vi "Data Archiving.vi"() -> ()   [LabVIEW 2009]
uses:
  lib/Apps/App Status Actions.ctl
  lib/Data Access Objects/Metadata/Persistant DAO Actions.ctl
  lib/Logging/LogFileType.ctl
  lib/MixedMode/Mixed Mode States.ctl
  lib/Launcher/Launcher Actions.ctl
  lib/Launcher/NoPanelAppTypes.ctl
  lib/Data Access Objects/Metadata/DAO Actions.ctl
  lib/MixedMode/Mixed Mode Archived State.ctl
  lib/Apps/Yes No Button.ctl
  lib/Global Data/Transactions/Dataset Type.ctl
  lib/Global Data/Transactions/Dataset Source.ctl
  lib/Global Data/Transactions/Dataset Transaction Id.ctl
  lib/Logging/Command or Stiffness Updates.ctl
  lib/Global Data/Jacobian Stiffness Column Id.ctl
  lib/Global Data/Jacobian Stiffness Column.ctl
  lib/MixedMode/Target Data.ctl
  lib/Global Data/Command Or Stiffness Update Type.ctl
  lib/Logging/Command or Stiffnness Record.ctl
  lib/Logging/Archive File Type.ctl
panel:
  out "current time":timestamp
  out "Step":string
  out "all stopped":bool
  out "Continuous Archive Buffer Size":i32(slide) scale=0.0..1000.0
  out "MixedModeStates":T1
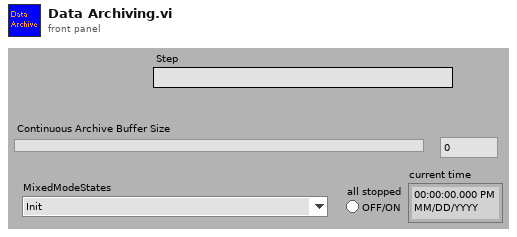
[diagram p1: front panel]
types:
  T1 = typedef "Mixed Mode States.ctl" = enum16{"Init", "Wait For DAQ", "Idle", "Start Initial Position", "Initial Position", "Start Initial Ramp", "Run Initial Ramp", "Start Iterative Stage", "Convergence Check", "Update Stiffness Jacobian", "Update Command", "Start Iterative Ramp", "Run Iterative Ramp", "Start Iterative Stabilize", "Iterative Stabilize", "Start Iterative Holding", "Iterative Holding", "Start Stabilize", "Stabilize", "Start Hold", "Holding", "Done", "Aborting", "Exit", "Nop"}
  T2 = typedef "Command or Stiffnness Record.ctl" = cluster{"Command || Stiffness Update":T3, "Records":string[]}
  T3 = typedef "Command or Stiffness Updates.ctl" = enum16{"Command Update", "Iterative Command Update", "Stiffness Update"}
  T4 = typedef "Command Or Stiffness Update Type.ctl" = cluster{"Target":T5[], "Stiffness":T6[], "Command || Stiffness Update":T3}
  T5 = typedef "Target Data.ctl" = cluster{"Displacements":dbl[], "Command Type":enum16{"<None>", "Displacement", "Force"}[], "Forces":dbl[]}
  T6 = typedef "Jacobian Stiffness Column.ctl" = cluster{"Id":T7, "Column":dbl[]}
  T7 = typedef "Jacobian Stiffness Column Id.ctl" = enum16{"dDx", "dDy", "dDz", "dRx", "dRy", "dRz"}
  T8 = typedef "Dataset Transaction Id.ctl" = cluster{"Dataset Source":T9, "Dataset Type":T10, "Hold":T11, "Volts":T11, "Tag":string}
  T9 = typedef "Dataset Source.ctl" = enum16{"LBCB 1", "LBCB 2", "Combined", "External Sensors"}
  T10 = typedef "Dataset Type.ctl" = enum16{"LVDT", "Load Cell", "Actuator Command", "Servo Error", "Displacement Command", "Displacement", "Force"}
  T11 = typedef "Yes No Button.ctl" = bool
  T12 = typedef "Mixed Mode Archived State.ctl" = cluster{"MixedModeStates":T1, "Step":string}
  T13 = typedef "Persistant DAO Actions.ctl" = enum16{"Init", "Get", "Set", "Load", "Save"}
  T14 = typedef "DAO Actions.ctl" = enum16{"Init", "Get", "Set"}
  T15 = typedef "Number Of LBCBs.ctl" = enum16{"1", "2"}
  T16 = typedef "App Parameters.ctl" = cluster{"Monitor Loop":T17, "Ramp Time":T17, "Log Loop":T17, "TCP to DAQ":T17, "Logging Directory":path, "Log File Size (MBytes)":i64, "Volt Logging Loop":T17, "2 LBCB Archiving Mode":bool}
  T17 = typedef "Timing Parameters.ctl" = cluster{"Interval":dbl, "Rate ":dbl}
  T18 = typedef "Archive File Type.ctl" = enum16{"LBCB1", "LBCB2", "ExternalSensors", "Combined"}
  T19 = typedef "App Status Actions.ctl" = enum16{"Init", "Get Status", "Running", "Control", "Autobalanced", "Data Acquisition", "Set App State", "DAQ Started", "Set LBCB State", "Set All", "Set Cont Logging", "Set Step Logging", "Set MM Logging", "Set Volt Logging", "Set DAQ Link"}
  T20 = typedef "LogFileType.ctl" = enum16{"Continuous", "Step", "Volts", "Offsets", "DLL  Errors", "Snapshot", "Commands", "StiffnessUpdates", "End List"}
  T21 = typedef "App Status.ctl" = cluster{"Running":bool, "Controlling L2":bool, "Autobalance L2":bool, "Data Acquisition":bool, " App State":T22, "DAQ Started":bool, "LBCB 1 State":T23, "LBCB 2 State":T23, "Controlling L1":bool, "Autobalance L1":bool, "Continuous Logging":bool, "Step Logging":bool, "Voltage Logging":bool, "Mixed Mode Logging":bool, "DAQ Link":bool}
  T22 = typedef "AppStates.ctl" = enum16{"Starting OM", "Initializing Displays", "Setting up Archiving", "Setting Up DAQ Channels", "Start DAQ", "DAQ Starting", "Controlling LBCBs", "Stopping OM"}
  T23 = typedef "Lbcb Control Loop States.ctl" = enum16{"Idle", "Start Selected", "Load Last Command", "Start Autobalancing", "Autobalancing", "Control Loop Initialized", "Control Enabled"}
  T24 = typedef "Network Parameters.ctl" = cluster{"Port Number":u16, "Notification Name":string, "Wait For Notification Timeout":i32}
  T25 = typedef "NoPanelAppTypes.ctl" = enum16{"NTCP Socket", "Data Archiving", "DAQ Link", "Control Loops", "Cmd Disp Diffs", "LBCB Data", "Limits", "Mixed Mode Widget", "Offsets"}
  T26 = typedef "Launcher Actions.ctl" = enum16{"Launch", "Stop All", "Stop", "Kill", "Running?", "Init"}
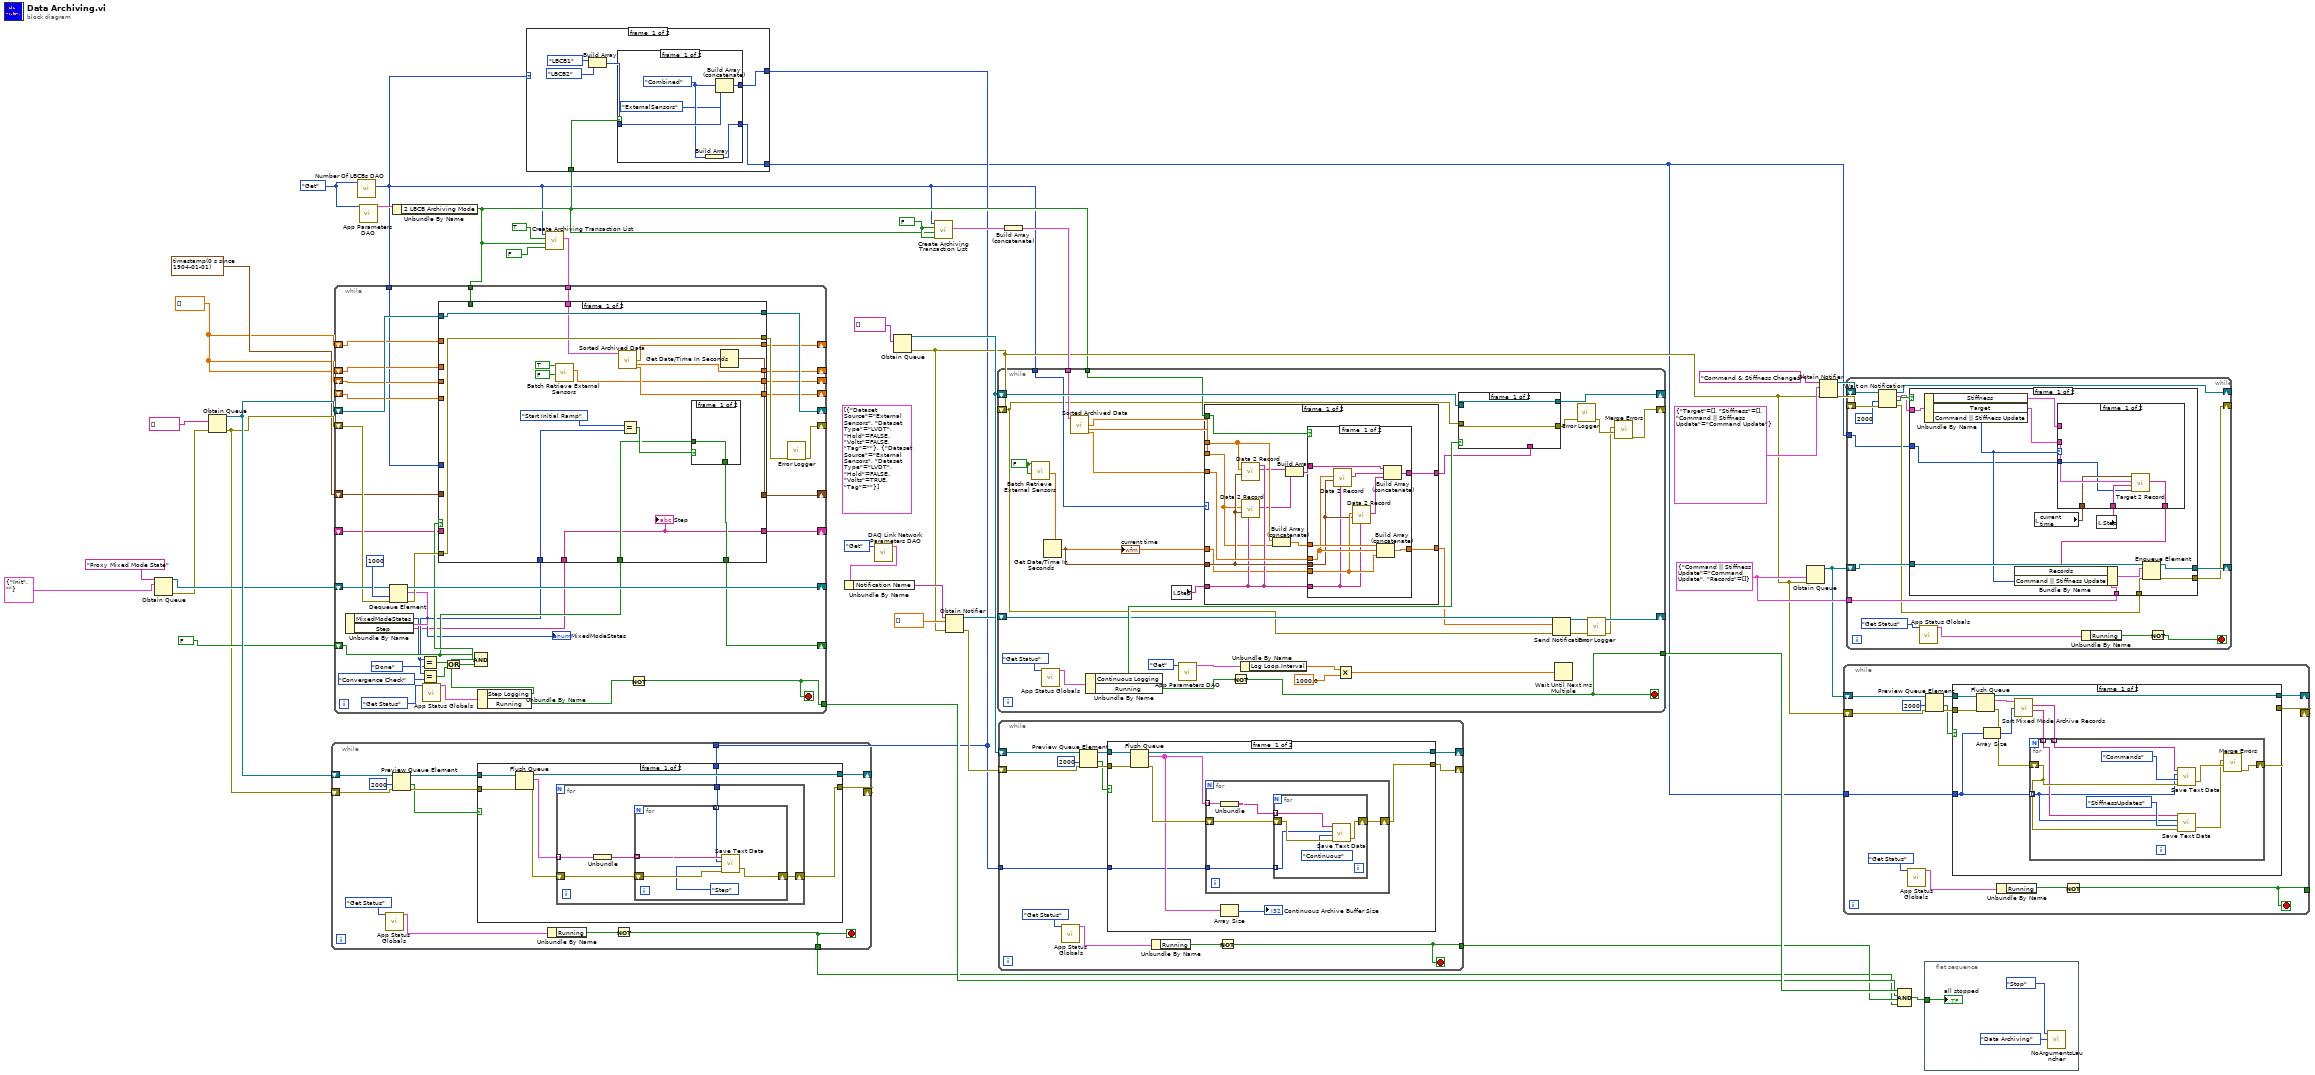
[diagram p0: block diagram]
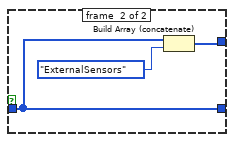
[diagram p2: hidden frame]
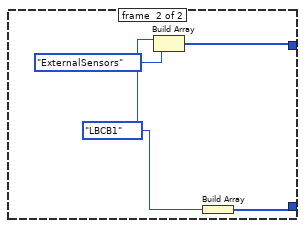
[diagram p3: hidden frame]
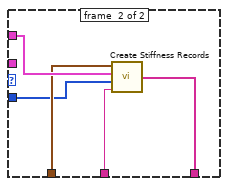
[diagram p5: hidden frame]
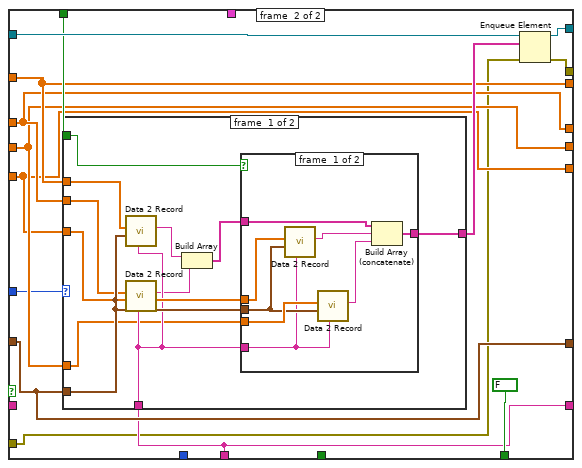
[diagram p9: hidden frame]
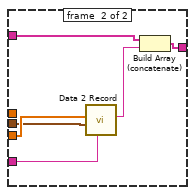
[diagram p10: hidden frame]
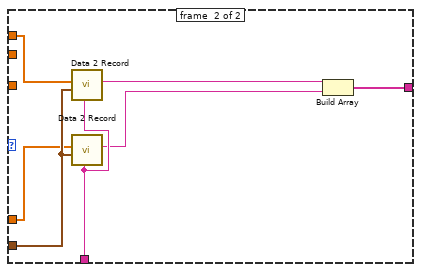
[diagram p11: hidden frame]
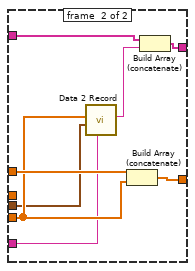
[diagram p13: hidden frame]
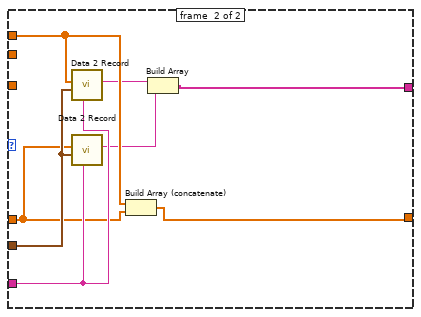
[diagram p14: hidden frame]
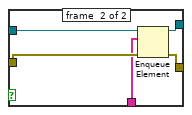
[diagram p15: hidden frame]
diagram:
  w7 = T2 {"Command || Stiffness Update"=enum."Command Update", "Records"=[]} ("Command || Stiffness Record")
  (unwired) T8[] [{"Dataset Source"=enum."External Sensors", "Dataset Type"=enum."LVDT", "Hold"=FALSE, "Volts"=FALSE, "Tag"=""}, {"Dataset Source"=enum."External Sensors", "Dataset Type"=enum."LVDT", "Hold"=FALSE, "Volts"=TRUE, "Tag"=""}] ("Transactions")
  w14 = T11 FALSE ("Hold")
  w21 = Persistant_DAO_Actions."Get" ("Actions")
  w25 = dbl[] [] ("Data")
  n1 = Obtain Queue(name (unnamed)="Proxy Mixed Mode State", element data type=T12 {"MixedModeStates"=enum."Init", "Step"=""} ("Mixed Mode Archived State")) -> (queue out=w38:refnum<queue>, error out=w37:errorcluster)  [unwired: 3 in, 1 out]
  n2 = Obtain Queue(element data type=string[] [] ("Records"), error in (no error)=w37) -> (queue out=w40:refnum<queue>, error out=w33:errorcluster)  [unwired: 2 in, 2 out]
  n3 = call "Number Of LBCBs DAO.vi"("Actions"=w21) -> ("Number of\nLBCBs Out"=w2:T15)  [unwired: 7 in, 3 out]
  n4 = call "App Parameters DAO.vi"("Actions"=w21) -> ("Application Timing and Logging Out"=w20:T16)  [unwired: 8 in, 2 out]
  n5 = Unbundle By Name(w20) -> ("2 LBCB Archiving Mode"=w4:bool)
  n6 = case shown="\"2\"" w2 {
    tunnel: w4 -> [w48 _]
    tunnel: [w44 w58] -> w3
    tunnel: [w43 w57] -> w1
    frame #0 {
      n7 = Build Array(Archive_File_Type."LBCB1" ("Archive File Type"), Archive_File_Type."LBCB2" ("element")) -> (w46:T18[])
      n8 = case shown="True" w48 {
        tunnel: w46 -> [w53 w56]
        tunnel: [w50 w54] -> w44
        tunnel: [w49 w56] -> w43
        frame #0 {
          w52 = Archive_File_Type."Combined" ("element")
          n9 = Build Array(w52) -> (w49:T18[])
          n10 = Build Array (concatenate)(w53, w52, Archive_File_Type."ExternalSensors" ("element")) -> (w50:T18[])
        }
        frame #1 {
          n11 = Build Array (concatenate)(w56, Archive_File_Type."ExternalSensors" ("element")) -> (w54:T18[])
        }
      }
    }
    frame #1 {
      w60 = Archive_File_Type."LBCB1" ("Archive File Type")
      n12 = Build Array(w60, Archive_File_Type."ExternalSensors" ("element")) -> (w58:T18[])
      n13 = Build Array(w60) -> (w57:T18[])
    }
  }
  n14 = while {
    shift-right: [w64] -> _
    shift-left: w40 -> [w67]
    shift-right: [w65] -> _
    shift-left: w33 -> [w66]
    tunnel: [w62] -> w29
    tunnel: w3 -> [w61]
    stop <- w62 stop-if-true
    n15 = call "App Status Globals.vi"("App Status Actions"=App_Status_Actions."Get Status") -> ("App Status Out"=w72:T21)  [unwired: 5 in, 9 out]
    n16 = Preview Queue Element(queue=w67, timeout in ms (-1)=2000, error in (no error)=w66) -> (queue out=w68:refnum<queue>, timed out?=w63:bool, error out=w69:errorcluster)  [unwired: 1 out]
    n17 = case shown="False" w63 {
      tunnel: w68 -> [w80 w92]
      tunnel: w69 -> [w79 w91]
      tunnel: [w78 w92] -> w64
      tunnel: [w76 w91] -> w65
      tunnel: w61 -> [w74 _]
      frame #0 {
        n18 = Flush Queue(queue=w80, error in (no error)=w79) -> (queue out=w78:refnum<queue>, remaining elements=w75:cluster{"Records":string[]}[], error out=w77:errorcluster)
        n19 = for {
          tunnel: w75 -> [w83] mode=indexing
          shift-right: [w84] -> w76
          shift-left: w77 -> [w85]
          tunnel: w74 -> [w81]
          n20 = Unbundle(w83) -> ("Records"=w82:string[])
          n21 = for {
            shift-right: [w88] -> w84
            shift-left: w85 -> [w90]
            tunnel: w82 -> [w87] mode=indexing
            tunnel: w81 -> [w86] mode=indexing
            n22 = call "Save Text Data.vi"("String"=w87, "Archive File Type"=w86, "LogFile Type"=LogFileType."Step", "error in"=w90) -> ("error out"=w88:errorcluster)  [unwired: 1 in, 1 out]
          }
        }
      }
      frame #1 {
      }
    }
    n23 = Unbundle By Name(w72) -> ("Running"=w73:bool)
    n24 = Not(x=w73) -> (.not. x?=w62:bool)
  }
  n25 = call "Create Archiving Transaction List.vi"("Volts Only"=FALSE ("Include Volts"), "Combined LBCBs"=w4, "Hold"=T11 TRUE, "Number of LBCBs"=w2) -> ("Transactions"=w15:T8[])  [unwired: 7 in]
  n26 = while {
    shift-right: [w128] -> _
    shift-left: w40 -> [w129]
    shift-right: [w126] -> _
    shift-left: w33 -> [w122]
    shift-right: [w123] -> _
    shift-left: w38 -> [w124]
    shift-right: [w118] -> _
    shift-left: FALSE -> [w115]
    tunnel: [w116] -> w31
    shift-right: [w114] -> _
    shift-left: timestamp(0 s since 1904-01-01) ("seconds since 1Jan1904") -> [w109]
    shift-right: [w113] -> _
    shift-left: w25 -> [w110]
    shift-right: [w112] -> _
    shift-left: w25 -> [w108]
    shift-right: [w111] -> _
    shift-left: w25 -> [w107]
    shift-right: [w104] -> _
    shift-left: _ -> [w103]
    shift-right: [w102] -> _
    shift-left: _ -> [w101]
    tunnel: w15 -> [w100]
    tunnel: w4 -> [w99]
    tunnel: w2 -> [w98]
    stop <- w116 stop-if-true
    n27 = Dequeue Element(queue=w124, timeout in ms (-1)=1000, error in (no error)=w122) -> (queue out=w123:refnum<queue>, element=w117:T12, error out=w121:errorcluster)  [unwired: 1 out]
    n28 = Unbundle By Name(w117) -> ("MixedModeStates"=w106:T1, "Step"=w105:string)
    "MixedModeStates" <- w106
    n29 = Equal?(x=w106, y=Mixed_Mode_States."Done") -> (x = y?=w96:bool)
    n30 = Equal?(x=w106, y=Mixed_Mode_States."Convergence Check") -> (x = y?=w95:bool)
    n31 = call "App Status Globals.vi"("App Status Actions"=App_Status_Actions."Get Status") -> ("App Status Out"=w131:T21)  [unwired: 5 in, 9 out]
    n32 = Or(x=w96, y=w95) -> (x .or. y?=w97:bool)
    n33 = Unbundle By Name(w131) -> ("Step Logging"=w120:bool, "Running"=w130:bool)
    n34 = Compound Arithmetic op=AND(w115, w120, w97) -> (w119:bool)
    n35 = case shown="True" w119 {
      tunnel: w129 -> [w148 w164]
      tunnel: w121 -> [w147 w151]
      tunnel: [w148 w163] -> w128
      tunnel: [w147 w162] -> w127
      tunnel: [w143 FALSE] -> w118
      tunnel: w106 -> [w146 _]
      tunnel: w115 -> [w142 _]
      tunnel: [w141 w160] -> w114
      tunnel: [w134 w156] -> w113
      tunnel: [w133 w155] -> w112
      tunnel: [w135 w154] -> w111
      tunnel: w110 -> [_ w156]
      tunnel: w109 -> [_ w160]
      tunnel: w108 -> [_ w155]
      tunnel: w107 -> [_ w154]
      tunnel: w105 -> [w140 w157]
      tunnel: [w140 w157] -> w104
      tunnel: w103 -> [_ _]
      tunnel: [w139 w153] -> w102
      tunnel: w101 -> [_ w153]
      tunnel: w100 -> [w138 _]
      tunnel: w99 -> [_ w159]
      tunnel: w98 -> [_ w152]
      frame #0 {
        n36 = call "Batch Retrieve External Sensors.vi"("Include Volts"=T11 FALSE, "Hold Data"=T11 TRUE) -> ("Data"=w135:dbl[])  [unwired: 8 in, 1 out]
        n37 = call "Sorted Archived Data.vi"("Transactions"=w138) -> ("LBCB 1"=w134:dbl[], "LBCB 2"=w133:dbl[], "Combined"=w139:dbl[])  [unwired: 10 in, 2 out]
        n38 = Equal?(x=Mixed_Mode_States."Start Initial Ramp", y=w146) -> (x = y?=w144:bool)
        n39 = case shown="True" w144 {
          selector: w144 -> [_ w150]
          tunnel: [w149 w150] -> w143
          tunnel: w142 -> [w149 _]
          frame #0 {
          }
          frame #1 {
          }
        }
        n40 = Get Date/Time In Seconds() -> (seconds since 1Jan1904=w141:timestamp)
        "Step" <- w140
      }
      frame #1 {
        n41 = case shown="\"1\"" w152 {
          tunnel: w156 -> [w171 w194]
          tunnel: w155 -> [w170 _]
          tunnel: w154 -> [w167 w190]
          tunnel: w153 -> [w174 _]
          tunnel: w159 -> [w175 _]
          tunnel: w160 -> [w173 w196]
          tunnel: w157 -> [w172 w195]
          tunnel: [w165 w191] -> w158
          frame #0 {
            n42 = call "Data 2 Record.vi"("Step"=w172, "Time Stamp"=w173, "Data"=w171) -> ("Records"=w169:string)  [unwired: 8 out]
            n43 = call "Data 2 Record.vi"("Step"=w172, "Time Stamp"=w173, "Data"=w170) -> ("Records"=w168:string)  [unwired: 8 out]
            n44 = Build Array(w169, w168) -> (w166:string[])
            n45 = case shown="True" w175 {
              tunnel: w174 -> [w183 _]
              tunnel: w173 -> [w181 w188]
              tunnel: w172 -> [w180 w187]
              tunnel: w167 -> [w182 w189]
              tunnel: w166 -> [w179 w186]
              tunnel: [w176 w184] -> w165
              frame #0 {
                n46 = call "Data 2 Record.vi"("Step"=w180, "Time Stamp"=w181, "Data"=w183) -> ("Records"=w178:string)  [unwired: 8 out]
                n47 = call "Data 2 Record.vi"("Step"=w180, "Time Stamp"=w181, "Data"=w182) -> ("Records"=w177:string)  [unwired: 8 out]
                n48 = Build Array (concatenate)(w179, w178, w177) -> (w176:string[])
              }
              frame #1 {
                n49 = call "Data 2 Record.vi"("Step"=w187, "Time Stamp"=w188, "Data"=w189) -> ("Records"=w185:string)  [unwired: 8 out]
                n50 = Build Array (concatenate)(w186, w185) -> (w184:string[])
              }
            }
          }
          frame #1 {
            n51 = call "Data 2 Record.vi"("Step"=w195, "Time Stamp"=w196, "Data"=w194) -> ("Records"=w193:string)  [unwired: 8 out]
            n52 = call "Data 2 Record.vi"("Step"=w195, "Time Stamp"=w196, "Data"=w190) -> ("Records"=w192:string)  [unwired: 8 out]
            n53 = Build Array(w193, w192) -> (w191:string[])
          }
        }
        n54 = Enqueue Element(queue=w164, element=w158, error in (no error)=w151) -> (queue out=w163:refnum<queue>, error out=w162:errorcluster)  [unwired: 2 out]
      }
    }
    n55 = Not(x=w130) -> (.not. x?=w116:bool)
    n56 = call "Error Logger.vi"("error in (no error)"=w127) -> ("error out"=w126:errorcluster)  [unwired: 1 in, 9 out]
  }
  n57 = call "DAQ Link Network Parameters DAO.vi"("Persistent DAO Actions"=DAO_Actions."Get" ("DAO Actions")) -> ("Network Parameters Out"=w24:T24)  [unwired: 3 in, 7 out]
  n58 = Unbundle By Name(w24) -> ("Notification Name"=w23:string)
  n59 = Obtain Queue(element data type=string[] [] ("Records")) -> (queue out=w42:refnum<queue>, error out=w5:errorcluster)  [unwired: 3 in, 2 out]
  n60 = call "Create Archiving Transaction List.vi"("Volts Only"=w14, "Combined LBCBs"=w4, "Hold"=w14, "Number of LBCBs"=w2) -> ("Transactions"=w16:T8[])  [unwired: 7 in]
  n61 = Obtain Notifier(name (unnamed)=w23, notification data type=dbl[] [] ("appended array"), error in (no error)=w5) -> (notifier out=w34:refnum<notifier>, error out=w19:errorcluster)  [unwired: 1 in, 1 out]
  n62 = while {
    shift-right: [w200] -> _
    shift-left: w42 -> [w203]
    shift-right: [w201] -> _
    shift-left: w19 -> [w202]
    tunnel: [w198] -> w30
    tunnel: w3 -> [w197]
    stop <- w198 stop-if-true
    n63 = call "App Status Globals.vi"("App Status Actions"=App_Status_Actions."Get Status") -> ("App Status Out"=w208:T21)  [unwired: 5 in, 9 out]
    n64 = Preview Queue Element(queue=w203, timeout in ms (-1)=2000, error in (no error)=w202) -> (queue out=w204:refnum<queue>, timed out?=w199:bool, error out=w205:errorcluster)  [unwired: 1 out]
    n65 = case shown="False" w199 {
      tunnel: w204 -> [w217 w229]
      tunnel: w205 -> [w216 w228]
      tunnel: [w215 w229] -> w200
      tunnel: [w212 w228] -> w201
      tunnel: w197 -> [w210 _]
      frame #0 {
        n66 = Flush Queue(queue=w217, error in (no error)=w216) -> (queue out=w215:refnum<queue>, remaining elements=w211:cluster{"Records":string[]}[], error out=w213:errorcluster)
        n67 = for {
          tunnel: w211 -> [w220] mode=indexing
          shift-right: [w221] -> w212
          shift-left: w213 -> [w222]
          tunnel: w210 -> [w218]
          n68 = Unbundle(w220) -> ("Records"=w219:string[])
          n69 = for {
            tunnel: w219 -> [w224] mode=indexing
            shift-right: [w225] -> w221
            shift-left: w222 -> [w227]
            tunnel: w218 -> [w223] mode=indexing
            n70 = call "Save Text Data.vi"("String"=w224, "Archive File Type"=w223, "LogFile Type"=LogFileType."Continuous", "error in"=w227) -> ("error out"=w225:errorcluster)  [unwired: 1 in, 1 out]
          }
        }
        n71 = Array Size(array=w211) -> (size(s)=→"Continuous Archive Buffer Size":i32)
      }
      frame #1 {
      }
    }
    n72 = Unbundle By Name(w208) -> ("Running"=w209:bool)
    n73 = Not(x=w209) -> (.not. x?=w198:bool)
  }
  n74 = Build Array (concatenate)(w16) -> (w13:T8[])
  n75 = while {
    shift-right: [w252] -> _
    shift-left: w42 -> [w253]
    shift-right: [w232] -> _
    shift-left: w5 -> [w234]
    shift-right: [w248] -> _
    shift-left: w34 -> [w249]
    tunnel: [w247] -> w32
    tunnel: w2 -> [w244]
    tunnel: w4 -> [w243]
    tunnel: w13 -> [w242]
    stop <- w247 stop-if-true
    w238 = T11 FALSE ("Hold Data")
    n76 = call "Batch Retrieve External Sensors.vi"("Include Volts"=w238, "Hold Data"=w238) -> ("Data No Volts"=w239:dbl[])  [unwired: 8 in, 1 out]
    n77 = call "App Status Globals.vi"("App Status Actions"=App_Status_Actions."Get Status") -> ("App Status Out"=w259:T21)  [unwired: 5 in, 9 out]
    n78 = Get Date/Time In Seconds() -> (seconds since 1Jan1904=w237:timestamp)
    "current time" <- w237
    n79 = call "Sorted Archived Data.vi"("Transactions"=w242) -> ("LBCB 1"=w241:dbl[], "LBCB 2"=w240:dbl[], "Combined"=w246:dbl[])  [unwired: 10 in, 2 out]
    n80 = Unbundle By Name(w259) -> ("Continuous Logging"=w250:bool, "Running"=w254:bool)
    n81 = local read "Step"() -> (w236:string)
    n82 = call "App Parameters DAO.vi"("Actions"=Persistant_DAO_Actions."Get") -> ("Application Timing and Logging Out"=w255:T16)  [unwired: 3 in, 7 out]
    n83 = case shown="\"1\"" w244 {
      tunnel: w241 -> [w268 w298]
      tunnel: w240 -> [w267 _]
      tunnel: w239 -> [w264 w293]
      tunnel: w246 -> [w273 _]
      tunnel: [w271 w294] -> w245
      tunnel: w243 -> [w274 _]
      tunnel: w237 -> [w270 w300]
      tunnel: w236 -> [w269 w299]
      tunnel: [w262 w295] -> w235
      frame #0 {
        n84 = call "Data 2 Record.vi"("Step"=w269, "Time Stamp"=w270, "Data"=w268) -> ("Records"=w266:string)  [unwired: 8 out]
        n85 = call "Data 2 Record.vi"("Step"=w269, "Time Stamp"=w270, "Data"=w267) -> ("Records"=w265:string)  [unwired: 8 out]
        n86 = Build Array (concatenate)(w268, w267) -> (w272:dbl[])
        n87 = Build Array(w266, w265) -> (w263:string[])
        n88 = case shown="True" w274 {
          tunnel: w273 -> [w282 _]
          tunnel: w272 -> [w284 w292]
          tunnel: [w283 w291] -> w271
          tunnel: w270 -> [w280 w289]
          tunnel: w269 -> [w279 w288]
          tunnel: w264 -> [w281 w290]
          tunnel: w263 -> [w278 w287]
          tunnel: [w275 w285] -> w262
          frame #0 {
            n89 = call "Data 2 Record.vi"("Step"=w279, "Time Stamp"=w280, "Data"=w282) -> ("Records"=w277:string)  [unwired: 8 out]
            n90 = call "Data 2 Record.vi"("Step"=w279, "Time Stamp"=w280, "Data"=w281) -> ("Records"=w276:string)  [unwired: 8 out]
            n91 = Build Array (concatenate)(w284, w282, w281) -> (w283:dbl[])
            n92 = Build Array (concatenate)(w278, w277, w276) -> (w275:string[])
          }
          frame #1 {
            n93 = call "Data 2 Record.vi"("Step"=w288, "Time Stamp"=w289, "Data"=w290) -> ("Records"=w286:string)  [unwired: 8 out]
            n94 = Build Array (concatenate)(w292, w290) -> (w291:dbl[])
            n95 = Build Array (concatenate)(w287, w286) -> (w285:string[])
          }
        }
      }
      frame #1 {
        n96 = call "Data 2 Record.vi"("Step"=w299, "Time Stamp"=w300, "Data"=w298) -> ("Records"=w297:string)  [unwired: 8 out]
        n97 = call "Data 2 Record.vi"("Step"=w299, "Time Stamp"=w300, "Data"=w293) -> ("Records"=w296:string)  [unwired: 8 out]
        n98 = Build Array (concatenate)(w298, w293) -> (w294:dbl[])
        n99 = Build Array(w297, w296) -> (w295:string[])
      }
    }
    n100 = Not(x=w254) -> (.not. x?=w247:bool)
    n101 = Unbundle By Name(w255) -> ("Log Loop.Interval"=w256:dbl)
    n102 = Multiply(x=w256, y=1000.0) -> (x*y=w258:dbl)
    n103 = case shown="True" w250 {
      tunnel: w253 -> [w302 w307]
      tunnel: w234 -> [w301 w306]
      tunnel: [w302 w305] -> w252
      tunnel: [w301 w304] -> w251
      tunnel: w235 -> [_ w303]
      frame #0 {
      }
      frame #1 {
        n104 = Enqueue Element(queue=w307, element=w303, error in (no error)=w306) -> (queue out=w305:refnum<queue>, error out=w304:errorcluster)  [unwired: 2 out]
      }
    }
    n105 = Send Notification(notification=w245, notifier=w249, error in (no error)=w234) -> (notifier out=w248:refnum<notifier>, error out=w233:errorcluster)
    n106 = Wait Until Next ms Multiple(millisecond multiple=w258) -> ()  [unwired: 1 out]
    n107 = call "Error Logger.vi"("error in (no error)"=w251) -> ("error out"=w231:errorcluster)  [unwired: 1 in, 9 out]
    n108 = call "Error Logger.vi"("error in (no error)"=w233) -> ("error out"=w230:errorcluster)  [unwired: 1 in, 9 out]
    n109 = call <vilib>:"Merge Errors.vi"("error in 3 (no error)"=w231, "error in 2 (no error)"=w230) -> ("error out"=w232:errorcluster)  [unwired: 5 in]
  }
  n110 = Obtain Queue(element data type=w7, error in (no error)=w5) -> (queue out=w6:refnum<queue>)  [unwired: 3 in, 2 out]
  n111 = Obtain Notifier(name (unnamed)="Command & Stiffness Changes", notification data type=T4 {"Target"=[], "Stiffness"=[], "Command || Stiffness Update"=enum."Command Update"} ("Command || Stiffness Update"), error in (no error)=w5) -> (notifier out=w9:refnum<notifier>, error out=w10:errorcluster)  [unwired: 1 in, 1 out]
  n112 = while {
    shift-right: [w311] -> _
    shift-left: w6 -> [w314]
    shift-right: [w312] -> _
    shift-left: w5 -> [w313]
    tunnel: [w309] -> _
    tunnel: w1 -> [w308]
    stop <- w309 stop-if-true
    n113 = call "App Status Globals.vi"("App Status Actions"=App_Status_Actions."Get Status") -> ("App Status Out"=w319:T21)  [unwired: 5 in, 9 out]
    n114 = Preview Queue Element(queue=w314, timeout in ms (-1)=2000, error in (no error)=w313) -> (queue out=w315:refnum<queue>, timed out?=w310:bool, error out=w316:errorcluster)  [unwired: 1 out]
    n115 = case shown="False" w310 {
      tunnel: w315 -> [w330 w341]
      tunnel: w316 -> [w329 w340]
      tunnel: [w328 w341] -> w311
      tunnel: [w326 w340] -> w312
      tunnel: w308 -> [w322 _]
      frame #0 {
        n116 = Flush Queue(queue=w330, error in (no error)=w329) -> (queue out=w328:refnum<queue>, remaining elements=w325:T2[], error out=w327:errorcluster)
        n117 = Array Size(array=w322) -> (size(s)=w321:i32)
        n118 = call "Sort Mixed Mode Archive Records.vi"("Raw Records"=w325, "Number of LBCBs"=w321) -> ("Command Records"=w324:string[], "Stiffness Records"=w323:string[])  [unwired: 3 in]
        n119 = for {
          shift-right: [w335] -> w326
          shift-left: w327 -> [w336]
          tunnel: w324 -> [w333] mode=indexing
          tunnel: w323 -> [w332] mode=indexing
          tunnel: w322 -> [w331] mode=indexing
          n120 = call "Save Text Data.vi"("String"=w332, "Archive File Type"=w331, "LogFile Type"=LogFileType."StiffnessUpdates", "error in"=w336) -> ("error out"=w334:errorcluster)  [unwired: 1 in, 1 out]
          n121 = call "Save Text Data.vi"("String"=w333, "Archive File Type"=w331, "LogFile Type"=LogFileType."Commands", "error in"=w336) -> ("error out"=w338:errorcluster)  [unwired: 1 in, 1 out]
          n122 = call <vilib>:"Merge Errors.vi"("error in 3 (no error)"=w338, "error in 2 (no error)"=w334) -> ("error out"=w335:errorcluster)  [unwired: 5 in]
        }
      }
      frame #1 {
      }
    }
    n123 = Unbundle By Name(w319) -> ("Running"=w320:bool)
    n124 = Not(x=w320) -> (.not. x?=w309:bool)
  }
  n125 = while {
    shift-right: [w349] -> _
    shift-left: w9 -> [w352]
    shift-right: [w343] -> _
    shift-left: w10 -> [w353]
    shift-right: [w345] -> _
    shift-left: w6 -> [w347]
    tunnel: w7 -> [w346]
    tunnel: w1 -> [w342]
    stop <- w354 stop-if-true
    n126 = Wait on Notification(notifier=w352, timeout in ms (-1)=2000, error in (no error)=w353) -> (notifier out=w349:refnum<notifier>, notification=w348:T4, timed out?=w350:bool, error out=w344:errorcluster)  [unwired: 1 in]
    n127 = case shown="False" w350 {
      tunnel: w348 -> [w371 _]
      tunnel: w347 -> [w369 w383]
      tunnel: w346 -> [w368 _]
      tunnel: [w365 w383] -> w345
      tunnel: w344 -> [w364 w382]
      tunnel: [w363 w382] -> w343
      tunnel: w342 -> [w358 _]
      frame #0 {
        n128 = Unbundle By Name(w371) -> ("Stiffness"=w361:T6[], "Target"=w370:T5[], "Command || Stiffness Update"=w362:T3)
        n129 = local read "current time"() -> (w359:timestamp)
        n130 = local read "Step"() -> (w360:string)
        n131 = case shown="\"Command Update\", Default" w362 {
          tunnel: w370 -> [w376 _]
          tunnel: [w375 w380] -> w366
          tunnel: w361 -> [_ w381]
          tunnel: w360 -> [w374 w378]
          tunnel: w359 -> [w373 w379]
          tunnel: w358 -> [w372 w377]
          frame #0 {
            n132 = call "Target 2 Record.vi"(8:w372, "Step"=w374, "Current Target In"=w376, "Time Stamp"=w373) -> ("String Records Out"=w375:string[])  [unwired: 7 in]
          }
          frame #1 {
            n133 = call "Create Stiffness Records.vi"("Step"=w378, 2:w377, "Stiffness Updates"=w381, "Timestamp"=w379) -> ("Records"=w380:string[])
          }
        }
        n134 = Bundle By Name(cluster=w368, "Records"=w366, "Command || Stiffness Update"=w362) -> (w367:T2)
        n135 = Enqueue Element(queue=w369, element=w367, error in (no error)=w364) -> (queue out=w365:refnum<queue>, error out=w363:errorcluster)  [unwired: 1 in, 1 out]
      }
      frame #1 {
      }
    }
    n136 = call "App Status Globals.vi"("App Status Actions"=App_Status_Actions."Get Status") -> ("App Status Out"=w356:T21)  [unwired: 5 in, 9 out]
    n137 = Unbundle By Name(w356) -> ("Running"=w357:bool)
    n138 = Not(x=w357) -> (.not. x?=w354:bool)
  }
  n139 = Compound Arithmetic op=AND(w32, w31, w30, w29) -> (w28:bool)
  n140 = flat-sequence {
    tunnel: w28 -> [w386]
    frame #0 {
      n141 = call "NoArgumentsLauncher.vi"("Application"=NoPanelAppTypes."Data Archiving", "Application Launcher Actions"=Launcher_Actions."Stop") -> ()  [unwired: 1 in, 9 out]
      "all stopped" <- w386
    }
  }
